vi "validate.vi"(8 "error in":errorcluster, 11 "PS Channel configuration":refnum<class "Power Supply Channel configuration.lvclass">) -> (0 "error out":errorcluster, 3 "PS Channel configuration out":refnum<class "Power Supply Channel configuration.lvclass">)   [LabVIEW 2025, in "Power Supply.lvlib" / "Power Supply Channel configuration.lvclass"]
doc: "Provides an interface for performing validation on a given configuration. Any children should define the behavior of this function to ensure that the configuration in memory can be used by the runtime class.Copyright 2017 National Instruments Corporation\n\nLicensed under the Apache License, Version 2.0 (the \"License\"); you may not use this file except in compliance with the License. You may obtain a copy of the License at http://www.apache.org/licenses/LICENSE-2.0\nUnless required by applicable law or agreed to in writing, software distributed under the License is distributed on an \"AS IS\" BASIS, WITHOUT WARRANTIES OR CONDITIONS OF ANY KIND, either express or implied. See the License for the specific language governing permissions and limitations under the License."
uses:
  Power Supply Channel configuration.lvclass
  Power Supply Channel configuration.lvclass/Power Supply Channel configuration.ctl
  Users/Public/Documents/Sandia National Labs/TSS Plugin/CEF.lvlibp
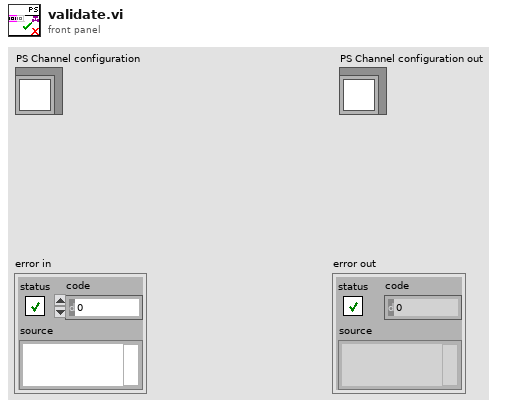
[diagram p1: front panel]
types:
  T1 = cluster{"Address":string, "SW Alias":string, "Enabled":bool, "Type":string, "Description":string}
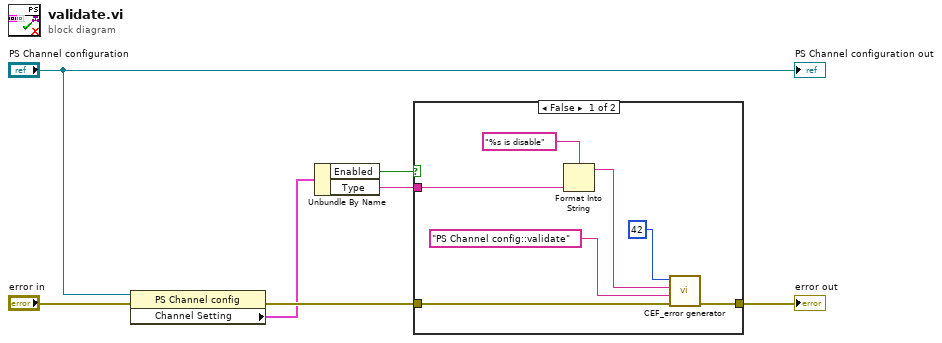
[diagram p0: block diagram]
diagram:
  n1 = property class="PS Channel config"(reference="PS Channel configuration", error in="error in") -> (error out=w5:errorcluster, "Channel Setting"=w3:T1)  [unwired: 1 out]
  n2 = Unbundle By Name(w3) -> ("Enabled"=w2:bool, "Type"=w1:string)
  n3 = case shown="False" w2 {
    tunnel: w5 -> [w14 w15]
    tunnel: [w13 w15] -> w7
    tunnel: w1 -> [w11 _]
    frame False {
      n4 = Format Into String(format string="%s is disable" ("append error message"), w11) -> (resulting string=w9:string)  [unwired: 2 in, 1 out]
      n5 = call "CEF_error generator.vi"("error in"=w14, "source"="PS Channel config::validate", "append error message"=w9, "error code (0)"=42) -> ("error out"=w13:errorcluster)  [unwired: 5 in]
    }
    frame True {
    }
  }
  "error out" <- w7
  "PS Channel configuration out" <- "PS Channel configuration"
